vi "Init.vi"() -> ()   [LabVIEW 2013]
uses:
  E:/Dropbox/ni/lvcef/github/lvcef/dotnet/LVCef/bin/Debug/Xilium.CefGlue.dll
  dotnet/LVCef/bin/Debug/Xilium.CefGlue.dll
panel:
  out "Numeric":i32
  out "error out":errorcluster
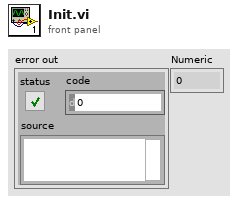
[diagram p1: front panel]
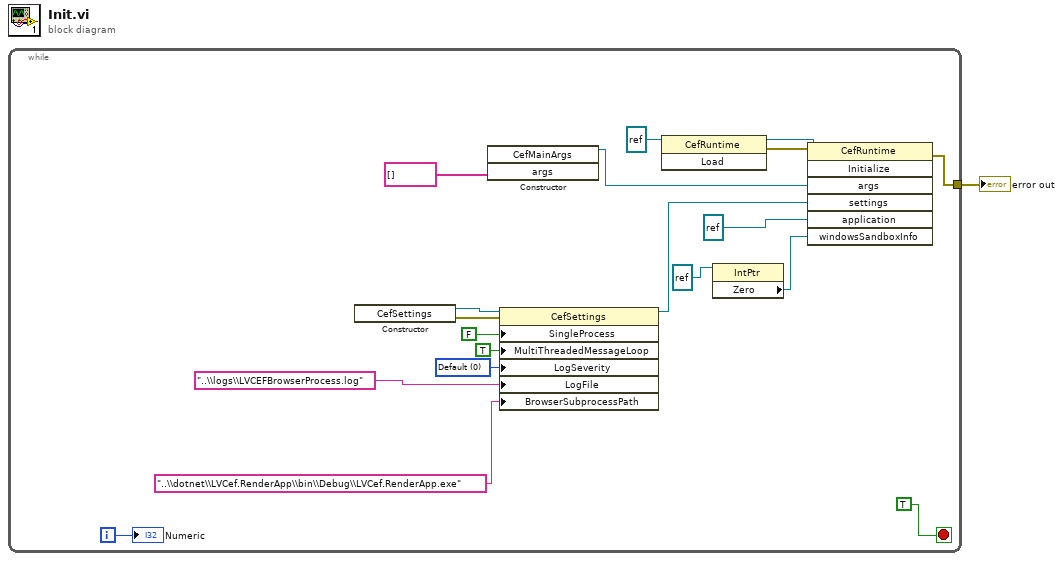
[diagram p0: block diagram]
diagram:
  n1 = while {
    tunnel: [w6] -> w1
    i -> [w5]
    stop <- TRUE stop-if-true
    w14 = 0 items=["Default"=0, "Verbose"=1, "Info"=2, "Warning"=3, "Error"=4, "ErrorReport"=5, "Disable"=99] ("LogSeverity")
    n2 = constructor class="CefSettings"() -> (reference out=w16:refnum<k24>, error out=w7:errorcluster)  [unwired: 3 in, 1 out]
    n3 = constructor class="CefMainArgs"("args"=string[] []) -> (reference out=w11:refnum<k24>)  [unwired: 3 in, 3 out]
    n4 = property class="CefSettings"(reference=w16, error in=w7, "SingleProcess"=FALSE, "MultiThreadedMessageLoop"=TRUE, "LogSeverity"=w14, "LogFile"="..\\logs\\LVCEFBrowserProcess.log", "BrowserSubprocessPath"="..\\dotnet\\LVCef.RenderApp\\bin\\Debug\\LVCef.RenderApp.exe") -> (reference out=w10:refnum<k24>)  [unwired: 1 out]
    n5 = invoke class="CefRuntime" method="Load"(reference=refnum<k24> refnum) -> (reference out=w19:refnum<k24>, error out=w18:errorcluster)  [unwired: 2 in, 1 out]
    n6 = property class="IntPtr"(reference=refnum<k24> refnum ("windowsSandboxInfo")) -> ("Zero"=w2:refnum<k24>)  [unwired: 1 in, 2 out]
    n7 = invoke class="CefRuntime" method="Initialize"(reference=w19, error in=w18, "args"=w11, "settings"=w10, "application"=refnum<k24> refnum, "windowsSandboxInfo"=w2) -> (error out=w6:errorcluster)  [unwired: 1 in, 6 out]
    "Numeric" <- w5
  }
  "error out" <- w1
